vi "Encoder.vi"() -> ()   [LabVIEW 2019]
doc: "This example shows how to configure, read values from, and reset an encoder.\n\nIt will display the encoder value, period, direction, and if the encoder is stopped.\n\nThis example expects a USB cable connected from your development PC to the Type B USB Jack (next to the power input) on the roboRIO."
uses:
  <vilib>/Rock Robotics/SystemInterfaces/DIO/FPGA_DIOChannel.ctl
  <vilib>/Rock Robotics/WPI/Encoder/WPI_EncoderType.ctl
  <vilib>/Rock Robotics/WPI/ThirdParty/Phoenix-LabVIEW/Motor Controller/Controls/CTRE_Phoenix_MotorControl_ControlMode.ctl
  <vilib>/Rock Robotics/WPI/Counter/WPI_CounterDigitalInputToDigitalSource.vi
panel:
  in  "Slide":dbl(slide) scale=-0.5..0.5
  in  "Device Number":u8=18
  out "Pitch Motor Dmd":dbl
  out "Value":bool
  in  "DIO Channel":T1
  in  "Number Samples to Average":u8=1 min=1 max=128
  in  "Invert Direction":bool=TRUE
  in  "Decoding Type":T2=enum."4x"
  in  "DistancePerCount":dbl=0.1
  in  "B Channel":T1=enum."DIO 1"
  in  "A Channel":T1
  out "Encoder Rate (distance/sec)":dbl
  out "Encoder Distance":dbl
  in  "Minimum Rate":dbl=20.0
  in  "stop":bool
  in  "Reset Encoder?":bool
  out "Encoder Alarm Status":string
  out "Encoder Direction":string
  # "Set these inputs before running."
  # "This can be set while running."
  # "Output information."
  # "Target"
  # "PITCH MOTOR    --- Any value over +/- 0.25 makes motor go..."
  # "This shows wiring for a generic quadrature encoder.  Some encoders may have Gnd labeled as Com.  Some may have +5V labeled as +VDC."
  # "Encoder\nB (white wire)---------\nGnd (black wire)------\n+5V (red wire)---------\nA (white wire)---------"
  # "roboRIO\nDIO-1  S\nDIO-0 \nDIO-0  V\nDIO-0  S"
  # "Encoder"
  # "Index"
  # "Gnd"
  # "+5V"
  # "B"
  # "A"
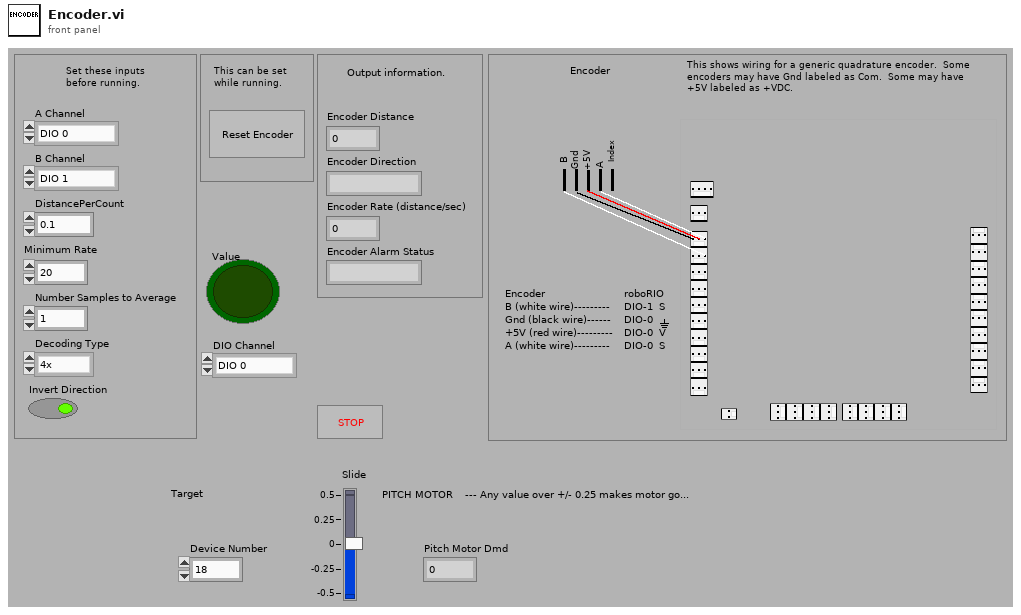
[diagram p1: front panel]
types:
  T1 = typedef "FPGA_DIOChannel.ctl" = enum8{"DIO 0", "DIO 1", "DIO 2", "DIO 3", "DIO 4", "DIO 5", "DIO 6", "DIO 7", "DIO 8", "DIO 9", "DIO MXP 0", "DIO MXP 1", "DIO MXP 2", "DIO MXP 3", "DIO MXP 4", "DIO MXP 5", "DIO MXP 6", "DIO MXP 7", "DIO MXP 8", "DIO MXP 9", "DIO MXP 10", "DIO MXP 11", "DIO MXP 12", "DIO MXP 13", "DIO MXP 14", "DIO MXP 15", "SPI Port CS1", "SPI Port CS2", "SPI Port CS3", "SPI Port MISO", "SPI Port MOSI", "Invalid"}
  T2 = typedef "WPI_EncoderType.ctl" = enum16{"1x", "2x", "4x"}
  T3 = typedef "WPI_MotorControlDeviceRef.ctl" = cluster{"DeviceStatus":errorcluster, "Type":T4, "PWM":cluster{"PWM Channel":T5, "DeadBand":T6}, "CAN":cluster{"Device Number":u8, "SetOutput VI Ref":variant, "GetOutput VI Ref":variant, "Enable VI Ref":variant, "Disable VI Ref":variant, "Data":variant}, "Invert":bool, "DIO PWM":cluster{"PWM \"Enable\" Channel":T5, "DIOChannel":T1, "PWM Rate":dbl}}
  T4 = typedef "WPI_MotorControlType.ctl" = enum16{"PWM", "CAN", "DIO PWM"}
  T5 = typedef "FPGA_DIOPWMChannel.ctl" = enum8{"PWM 0", "PWM 1", "PWM 2", "PWM 3", "PWM 4", "PWM 5", "PWM 6", "PWM 7", "PWM 8", "PWM 9", "PWM MXP 0", "PWM MXP 1", "PWM MXP 2", "PWM MXP 3", "PWM MXP 4", "PWM MXP 5", "PWM MXP 6", "PWM MXP 7", "PWM MXP 8", "PWM MXP 9", "Invalid"}
  T6 = typedef "WPI_PWMDeadband.ctl" = cluster{"Name":string, "maxPositivePwm":i32, "minPositivePwm":i32, "centerPwm":i32, "maxNegativePwm":i32, "minNegativePwm":i32, "angularRange":u16}
  T7 = typedef "WPI_DigitalInputDevRef.ctl" = cluster{"DevStatus":errorcluster, "DIO Channel":T1}
  T8 = typedef "FPGA_CounterEncoderSourceConvertionLVSourceType.ctl" = cluster{"DevStatus":errorcluster, "AnalogTriggerMode?":bool, "DigitalMode":cluster{"DIO Channel":T9}, "AnalogTriggerMode":cluster{"AnalogTriggerIndex":T10, "OutputType":T11}}
  T9 = typedef "FPGA_DIODigitalSourceChannel.ctl" = enum8{"DIO 0", "DIO 1", "DIO 2", "DIO 3", "DIO 4", "DIO 5", "DIO 6", "DIO 7", "DIO 8", "DIO 9", "DIO MXP 0", "DIO MXP 1", "DIO MXP 2", "DIO MXP 3", "DIO MXP 4", "DIO MXP 5", "DIO MXP 6", "DIO MXP 7", "DIO MXP 8", "DIO MXP 9", "DIO MXP 10", "DIO MXP 11", "DIO MXP 12", "DIO MXP 13", "DIO MXP 14", "DIO MXP 15", "SPI Port CS1", "SPI Port CS2", "SPI Port CS3", "SPI Port MISO", "SPI Port MOSI", "Disabled"}
  T10 = typedef "FPGA_AnalogTriggerIndex.ctl" = enum8{"Trig 0", "Trig 1", "Trig 2", "Trig 3", "Trig 4", "Trig 5", "Trig 6", "Trig 7", "Invalid"}
  T11 = typedef "FPGA_AnalogTriggerOutType.ctl" = enum16{"InWindow", "TriggerState", "Rising", "Falling"}
  T12 = typedef "WPI_EncoderDevRef.ctl" = cluster{"DevStatus":errorcluster, "EncoderIndex":T13, "CounterIndex":T14, "DistancePerCount":dbl, "Decoding Type":T2}
  T13 = typedef "FPGA_EncoderIdx.ctl" = enum8{"Enc 0", "Enc 1", "Enc 2", "Enc 3", "Enc 4", "Enc 5", "Enc 6", "Enc 7", "Invalid"}
  T14 = typedef "FPGA_CounterCtrSystemIndex.ctl" = enum8{"Ctr 0", "Ctr 1", "Ctr 2", "Ctr 3", "Ctr 4", "Ctr 5", "Ctr 6", "Ctr 7", "Invalid"}
  T15 = typedef "CTRE_Phoenix_MotorControl_ControlMode.ctl" = u16
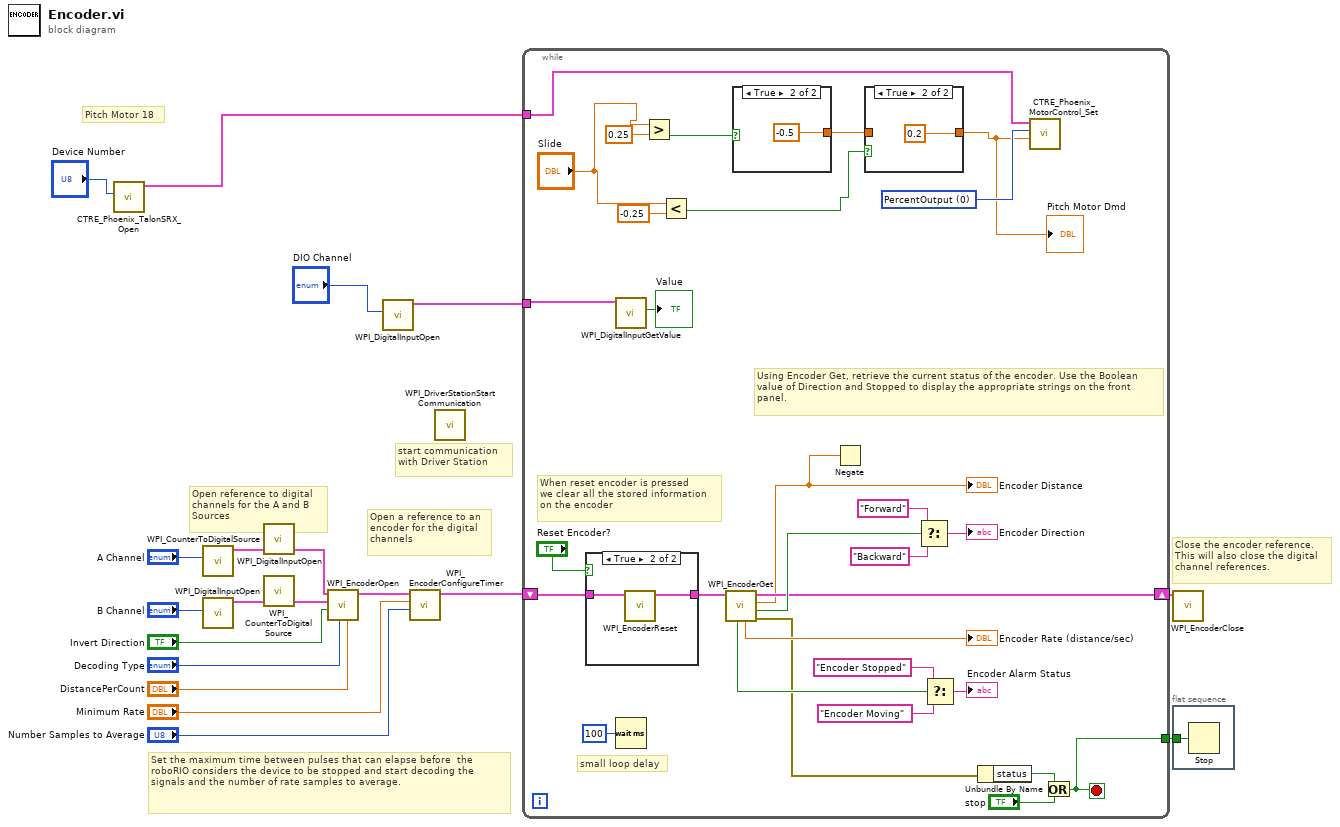
[diagram p0: block diagram]
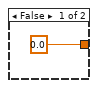
[diagram p3: hidden frame]
diagram:
  # "Pitch Motor 18"
  # "start communication with Driver Station"
  # "Close the encoder reference.\nThis will also close the digital \nchannel references."
  # "Set the maximum time between pulses that can elapse before  the roboRIO considers the device to be stopped and start decoding the signals and the number of rate samples to average."
  # "Open a reference to an\nencoder for the digital \nchannels"
  # "Open reference to digital \nchannels for the A and B\nSources"
  n1 = call <vilib>:"CTRE_Phoenix_TalonSRX_Open.vi"("Device Number"="Device Number") -> ("CAN Talon SRX Ref"=w1:T3)  [unwired: 9 in, 1 out]
  n2 = call <vilib>:"WPI_DigitalInputOpen.vi"("DIO Channel"="A Channel") -> ("DigitalInputDevRef"=w16:T7)  [unwired: 1 in, 9 out]
  n3 = call <vilib>:"WPI_DigitalInputOpen.vi"("DIO Channel"="B Channel") -> ("DigitalInputDevRef"=w17:T7)  [unwired: 1 in, 9 out]
  n4 = call-poly <vilib>:"WPI_CounterToDigitalSource.vi"("DigitalInputDevRef"=w16) -> ("Digital Source"=w15:T8)  [unwired: 6 out]
  n5 = call-poly <vilib>:"WPI_CounterToDigitalSource.vi"("DigitalInputDevRef"=w17) -> ("Digital Source"=w18:T8)  [unwired: 6 out]
  n6 = call <vilib>:"WPI_EncoderOpen.vi"("DistancePerCount"="DistancePerCount", "Decoding Type"="Decoding Type", "Invert Direction (False)"="Invert Direction", "BSource"=w18, "ASource"=w15) -> ("EncoderDevRef"=w8:T12)  [unwired: 3 in, 3 out]
  n7 = call <vilib>:"WPI_DigitalInputOpen.vi"("DIO Channel"="DIO Channel") -> ("DigitalInputDevRef"=w3:T7)  [unwired: 9 in, 1 out]
  n8 = call <vilib>:"WPI_EncoderConfigureTimer.vi"("Number Samples to Average"="Number Samples to Average", "Minimum Rate"="Minimum Rate", "EncoderDevRef"=w8) -> ("EncoderDevRef"=w9:T12)  [unwired: 1 in, 7 out]
  n9 = call <vilib>:"WPI_DriverStationStart Communication.vi"() -> ()  [unwired: 3 in, 9 out]
  n10 = while {
    shift-right: [w42] -> w19
    shift-left: w9 -> [w47]
    tunnel: [w40] -> w5
    tunnel: w3 -> [w31]
    tunnel: w1 -> [w27]
    stop <- w40 stop-if-true
    w28 = T15 0 items=["PercentOutput"=0, "Position"=1, "Velocity"=2, "Current"=3, "Follower"=5, "MotionProfile"=6, "MotionMagic"=7, "MotionProfileArc"=10, "Disabled"=15] ("Control Mode")
    # "small loop delay"
    # "Using Encoder Get, retrieve the current status of the encoder. Use the Boolean value of Direction and Stopped to display the appropriate strings on the front panel."
    # "When reset encoder is pressed\nwe clear all the stored information\non the encoder"
    n11 = case shown="True" "Reset Encoder?" {
      tunnel: w47 -> [w54 w56]
      tunnel: [w54 w55] -> w45
      frame False {
      }
      frame True {
        n12 = call <vilib>:"WPI_EncoderReset.vi"("EncoderDevRef"=w56) -> ("EncoderDevRef"=w55:T12)  [unwired: 1 in, 9 out]
      }
    }
    n13 = call <vilib>:"WPI_DigitalInputGetValue.vi"("DigitalInputDevRef"=w31) -> ("Value"=→"Value":bool)  [unwired: 8 in, 2 out]
    n14 = Wait (ms)(milliseconds to wait=u32 100) -> ()  [unwired: 1 out]
    n15 = Greater?(x="Slide", y=0.25) -> (0:w23:bool)
    n16 = Less?(x="Slide", y=-0.25) -> (x < y?=w22:bool)
    n17 = call <vilib>:"WPI_EncoderGet.vi"("EncoderDevRef"=w45) -> ("error out"=w38:errorcluster, "Direction"=w44:bool, "Distance"=w20:dbl, "EncoderDevRef"=w42:T12, "Rate"=→"Encoder Rate (distance/sec)":dbl, "Stopped"=w43:bool)  [unwired: 1 in, 4 out]
    "Encoder Distance" <- w20
    n18 = case shown="True" w23 {
      tunnel: [0.0 -0.5] -> w29
      frame False {
      }
      frame True {
      }
    }
    n19 = Negate(x=w20) -> ()  [unwired: 1 out]
    n20 = case shown="True" w22 {
      tunnel: w29 -> [w50 _]
      tunnel: [w50 0.2] -> w21
      frame False {
      }
      frame True {
      }
    }
    "Pitch Motor Dmd" <- w21
    n21 = Select(t="Forward", s=w44, f="Backward") -> (s? t:f=→"Encoder Direction":string)
    n22 = Select(t="Encoder Stopped", s=w43, f="Encoder Moving") -> (s? t:f=→"Encoder Alarm Status":string)
    n23 = Unbundle By Name(w38) -> ("status"=w36:bool)
    n24 = call <vilib>:"CTRE_Phoenix_MotorControl_Set.vi"("Output"=w21, "Control Mode"=w28, "PhoenixMotorControlDevRef"=w27) -> ()  [unwired: 7 in, 2 out]
    n25 = Or(x=w36, y="stop") -> (x .or. y?=w40:bool)
  }
  n26 = call <vilib>:"WPI_EncoderClose.vi"("EncoderDevRef"=w19) -> ()  [unwired: 2 in, 9 out]
  n27 = flat-sequence {
    tunnel: w5 -> [w57]
    frame #0 {
      n28 = Stop(stop? (T)=w57) -> ()
    }
  }
